vi "SPC_configure_memory.vi"(6 "No of Routing\nChannels":i16(ring)=12 items=["1"=1, "2"=2, "3"=3, "4"=4, "5"=5, "6"=6, "7"=7, "8"=8, "9"=9, "10"=10, "11"=11, "12"=12, "13"=13, "14"=14, "15"=15, "16"=16], 8 "Error In":errorcluster, 9 "ADC Resolution [exponent]":T2=7 items=["-1"=255, "1"=0, "4"=2, "16"=4, "64"=6, "256"=8, "1024"=10, "4096"=12], 10 "Module No":i16=-1 min=-1 max=7 step=1, 11 "DLL Path":path) -> (0 "Error Out":errorcluster, 2 "Module No":i16, 3 "DLL Path":path, 4 "#CurvesPerBank":i32, 5 "SPCMemConfig":T1={"Max Block No"=0, "Blocks Per Frame"=0, "Frames Per Page"=1, "Maxpage"=1, "Block Length"=1} {"Frames Per Page" min=1 step=1; "Maxpage" min=1; "Blocks Per Frame" min=1 step=1})   [LabVIEW 2023]
doc: "adc_resolution: ADC resolution (-1*,6,8,10,12 additionally 0,2,4 for SPC 830/140/930/15x/131/160) \n * With adc_resolution = -1 the procedure 'mem_info' is filled with the current values disregarding 'no_of_routing_bits'. \nno_of_routing_bits: number of routing bits (0 - 3 for SPC-130) (0 - 7 for SPC 6x0/140/15x/131/160) (0 - 14 for SPC-7xx(830) modules)\n\nThe procedure configures the memory of SPC module 'mod_no' depending on the specified ADC resolution, the module type and the number of detector channels (if a router is used). The action is done for normal operation modes. In FIFO modes the procedure sets hardware defined fixed values to ADC and no_of_routing_bits. In Scan modes the procedure does not configure the memory and should be called with 'adc_resolution' = -1 to get the current state of the DLL SPCMemConfig structure ( after setting scan parameters).\nIf 'mod_no' = -1, memory will be configured on all SPC modules which are actually in use.\nThe procedure has to be called before the first access to the SPC memory or before a measurement is started and always after setting ADC resolution parameter value. The memory configuration determines in which part of SPC memory the measurement data is recorded (see also SPC_set_page).\nThe SPC memory is interpreted as a set of 'pages'. One page contains a number of 'blocks'. \nOne block contains one decay curve. The number of points per block (per curve) is defined by the ADC resolution. The number of blocks per page depends on the number of points per block and on the number of detector channels (PointsX and PointsY)\nIn the scanning modes of the SPC-7/8/9/140/15x/160, a page contains a number of 'frames' (normally 1). Each frame contains a number of blocks. The number of blocks per page depends on the number of points per block and on the number of detector channels (PointsX and PointsY) and on the scanning parameters (pixels per line and lines per frame).\nThe differences between the modules are listed below.\nSPC-13x/6x0/15x/160 modules:\nThe length of the recorded curves is determined by the ADC resolution and can range from 64( 0 for SPC-15x/131/160) to 4096. Therefore, the number of complete measurement data sets (or 'pages') depends on the ADC resolution and the number of routing bits used.\nSPC-13x/6x0/15x/160 modules in the Histogram modes:\nThe length of the recorded curves is determined by the ADC resolution and can range from 64 ( 0 for SPC-15x/131/160) to 4096. Therefore, the number of complete measurement data sets (or 'pages') depends on the ADC resolution and the number of routing bits used.\nSPC-13x/6x0/830/140/15x/160/930 modules in the Fifo modes:\nThe module memory is configured as a FIFO memory - there are no curves and pages. Instead, a stream of collected photons is written to the fifo. A SPC_configure_memory function call is not required.\nSPC-7x0/830/140/15x/131/160 modules, Normal operation modes:\nThe length of the recorded curves is determined by the ADC resolution and can range from 0( SPC-830 and other) or 64( only SPC-7x0) to 4096. Therefore, the number of complete \nmeasurement data sets (or 'pages') depends on the ADC resolution and the number of routing \nbits used.\nSPC-7x0/830/140/15x/160/930 modules, Scanning modes:\nThe Memory configuration is not done not by SPC_configure_memory. Instead, the memory is configured by setting the parameters: \nADC_RESOLUTION - defines block_length,\nSCAN_SIZE_X, SCAN_SIZE_Y - defines blocks_per_frame\nSCAN_ROUT_X, SCAN_ROUT_Y - defines frames_per_page\nHowever, after setting these parameters SPC_configure_memory should be called with 'adc_resolution' = -1 to get the current state of the DLL SPCMemConfig structure.\nTo ensure correct access to the curves in the memory by the memory read/write functions, the SPC_configure_memory function loads a structure of the type SPCMemConfig with the values listed below:\nlong max_block_no total number of blocks (=curves) in the memory (per memory bank for the SPC- 6x0(13x/15x/160))\nlong blocks_per_frame Number of blocks (=curves) per frame\nlong frames_per_page Number of frames per page\nlong maxpage max number of pages to use in a measurement\nshort block_length Number of curve points16-bits words per block (curve)\nPossible operation modes for the SPC modules are defined in the spcm_def.h file. \nThe operation mode can be changed by setting the parameter MODE.\n\ninfo@becker-hickl"
uses:
  SPC_Controls/ConfigMem.ctl
  SPC_Controls/ADCResolution.ctl
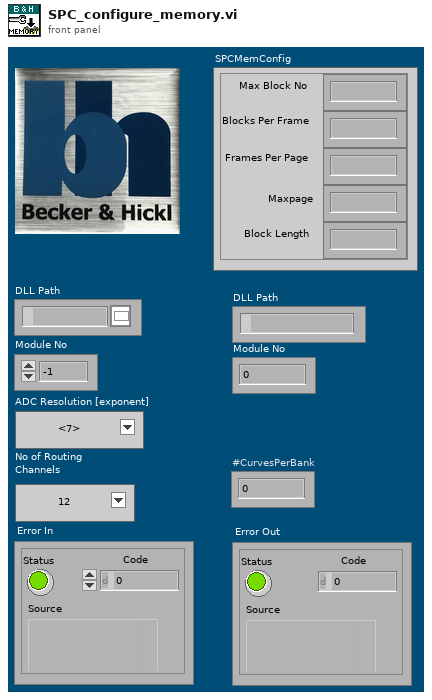
[diagram p1: front panel]
types:
  T1 = typedef "ConfigMem.ctl" = cluster{"Max Block No":i32, "Blocks Per Frame":i32, "Frames Per Page":i32, "Maxpage":i32, "Block Length":i32}
  T2 = typedef "ADCResolution.ctl" = i16
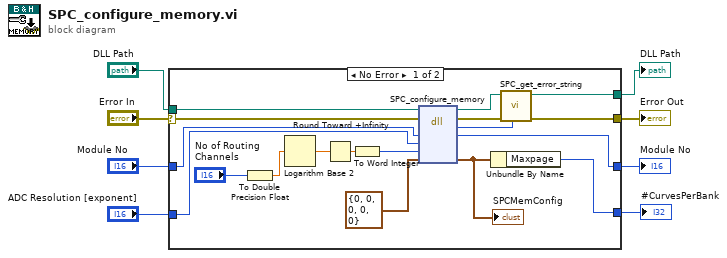
[diagram p0: block diagram]
diagram:
  n1 = case shown="No Error" "Error In" {
    selector: "Error In" -> [w22 w28]
    tunnel: "DLL Path" -> [w25 w29]
    tunnel: [w17 w28] -> w7
    tunnel: [w18 w29] -> w3
    tunnel: [w19 w27] -> w5
    tunnel: "Module No" -> [w23 w27]
    tunnel: "ADC Resolution [exponent]" -> [w13 _]
    tunnel: [w11 _] -> w1
    frame No Error {
      n2 = To Double Precision Float(number="No of Routing\nChannels") -> (double precision float=w12:dbl)
      n3 = Logarithm Base 2(1:w12) -> (0:w15:dbl)
      n4 = Round Toward +Infinity(x=w15) -> (ceil(x): smallest int >= x=w16:dbl)
      n5 = To Word Integer(number=w16) -> (16bit integer=w9:i16)
      n6 = dll-call lib="D:/spcm/lib/lab_view/lv10.0/spcm32.dll" fn="SPC_configure_memory"(path in=w25, error in=w22, "mod_no"=w23, "adc_resolution"=w13, "no_of_routing_bits"=w9, "mem_info"=T1 {"Max Block No"=0, "Blocks Per Frame"=0, "Frames Per Page"=0, "Maxpage"=0, "Block Length"=0} ("SPC Memory Config")) -> (path out=w26:path, error out=w21:errorcluster, "return type"=w20:i16, "mod_no"=w19:i16, "mem_info"=w14:T1)  [unwired: 3 in]
      "SPCMemConfig" <- w14
      n7 = Unbundle By Name(w14) -> ("Maxpage"=w11:i32)
      n8 = call "SPC_get_error_string.vi"("ErrorID"=w20, "Error In"=w21, "DLL Path"=w26) -> ("Error Out"=w17:errorcluster, "DLL Path"=w18:path)  [unwired: 6 in, 1 out]
    }
    frame Error {
    }
  }
  "Error Out" <- w7
  "DLL Path" <- w3
  "Module No" <- w5
  "#CurvesPerBank" <- w1
